vi "RSSI_Scanning.vi"() -> ()   [LabVIEW 2017]
uses:
  <vilib>/Instr/_visa.llb/VISA Configure Serial Port (Instr).vi
  Global Stop Variable.vi
  <vilib>/addons/_office/excel.llb/Excel Easy Table (str).vi
  <vilib>/Utility/NIReport.llb/NI_report.lvclass
  <vilib>/addons/_office/NI_ReportGenerationToolkit.lvlib
  <vilib>/Utility/NIReport.llb/Excel/NI_Excel.lvclass
panel:
  out "source":string
  out "code":i32
  out "error out":errorcluster
  out "STATUS":string
  in  "STOP":bool
  in  "Mode":T1(radio)
  out "Selesai Download":bool
  out "error out 2":errorcluster
  out "SSID 3":string
  out "SSID array":string[](array[string])
  out "dbm array":i32[](array[numeric])
  out "Color Box 3":u32(colorbox)=56508
  in  "Tab Control":T2(tab)
  in  "Tab Control 5":T3(tab)
  out "Background 8":string="Seiring dengan perkembangan teknologi informasi dan komunikasi yang pesat, jumlah pengguna internet di dunia mencapai 4,66 miliyar pada bulan januari tahun 2021 (Menurut hasil survey Hootsuite). Melihat data tersebut dapat disimpulkan bahwa akses internet sangat diminati dan menjadi kebutuhan utama oleh pengguna layanan internet [1]. Ada beberapa cara untuk mengakses internet yaitu dengan, Satellite, Celululer, Dial-Up, DSL, Cable, dan Wireless. WiFi, Berdasarkan IEEE 802.11 adalah sepesifikasi protokol jaringan lokal , dimana memungkinkan untuk mengakses internet dalam area yang terbatas menggunakan titik akses jaringan nirkabel atau dikenal dengan access point.  \nAccess point adalah perangkat jaringan yang berguna untuk membuat jaringan nirkabel yang sifatnya lokal dan berfungsi sebagai pintu gerbang bagi pengguna jaringan nirkabel untuk masuk ke dalam jaringan lokal.  Pada access point terdapat antena pengirim dan penerima sinyal, antena ini bertugas untuk memancarkan dan menerima sinyal dari clien server ataupun menuju clien server untuk bisa memancarkan sinyal WiFi. Dalam proses pengiriman dan penerimaan tersebut ada beberapa sistem untuk meningkatkan proses pengiriman dan penerimaan sinyal pada access point, yaitu menggunakan sistem MIMO pada access point, sehingga proses pengiriman dan penerimaan sinyal dapat meningkatkan kapasitas kanal atau jumlah aliran spasial [2][3].\n\nProses pengiriman dan penerimaan sinyal pada access point  dapat dilihat kekuatan sinyalnya dari parameter RSSI. Dalam literatur, [4] menyatakan bahwa RSSI merupakan parameter yang digunakan untuk mengukur indikator kekuatan sinyal yang diterima oleh sebuah access point. Dalam literatur, [5][6][7][8] parameter RSSI dimanfaatkan untuk membandingan kekuatan sinyal dan menganalisa hasil pengukuran RSSI terhadap access poin, jarak, dan ketinggian yang berbeda, dengan menggunakan perangkat lunak WiFi analyzer. Pada studi literatur tersebut terdapat dua kekurangan, yang pertama, dalam studi literatur terdahulu hanya menganalisa pengukuran RSSI terhadap variabel jarak dan tinggi terhadap acces point belum ada yang menganalisa pengukuran RSSI terhadap variabel polarisasi antena, dan yang kedua mengenai alat ukur yang digunakan oleh studi literatur, yaitu WiFi analyzer yang digunakan tidak memiliki fitur riwayat tercatat.\n\nBerdasarkan pemaparan di atas, maka dari itu diusulkan judul tugas akhir    \"Perancangan Wifi Analyzer Berbasis LabVIEW Untuk Membandingkan Parameter RSSI Pada Antena Access Point Sistem MIMO\".    Penelitian eksperimen ini diharapakan, pertama membuat alat ukur WiFi analyzer menggunakan NodeMCU  basis LabVIEW dengan fitur riwayat tercatat ke database, keterbukaan akses informasi dalam memperoleh parameter RSSI dan kemudahan komunikasi antar perangkat keras dengan perangkat lunak . Kedua, mengetahui ketepatan pengukuran kekuatan sinyal terima pada acces poin antena sistem MIMO menggunakan alat ukur yang telah dibuat. Ketiga, menganalisis pengaruh parameter RSSI dengan merubah variabel polarisasi pada antena access point sistem MIMO.\n\n"
  out "Background 7":string="Pemanas memiliki peran penting dalam proses industri, terutama industri kimia, yaitu untuk meningkatkan efisiensi proses dan menghasilkan kualitas produk yang baik. Salah satu jenis pemanas di industri kimia yang banyak digunakan adalah pemanas tangki berpengaduk. Pemanas tangki berpengaduk terdiri dari beberapa bagian, salah satunya adalah heater yang digunakan sebagai pemanas untuk mengubah bahan baku menjadi produk yang lebih bernilai guna. (N. I. Septiani, dkk, 2017)\n\nMasalah yang sering dihadapi dalam proses tersebut adalah keakuratan suhu pada tangki pemanas. Agar suhu tangki tersebut mencapai titik setel dengan kecepatan respons dan akurasi yang tinggi, maka diperlukan sebuah pengendali. (N. I. Septiani, dkk, 2017) Pengendali PID merupakan salah satu jenis pengendali yang paling banyak digunakan pada industri kimia dan industri yang memproduksi berbagai minuman seperti minuman coklat, susu, dan berbagai produk minuman lainnya. (A. Ramadhani, 2016) Untuk menghadapi tantangan industri tersebut, mahasiswa Diploma IV harus menguasai ilmu dan teknologi mengenai pengendali suhu pemanas tangki berpengaduk berbasis PID. \n\nMenurut Herman Dwi Surjono, media pembelajaran adalah program pembelajaran yang berisi teks, gambar, animasi, simulasi secara terpadu untuk mencapai tujuan pembelajaran. Media pembelajaran interaktif adalah program pembelajaran dimana pengguna secara aktif berinteraksi dengan program. Media pembelajaran interaktif memiliki ciri yaitu dapat mengontrol dan berinteraksi secara dinamis. Media pembelajaran interaktif dapat menumbuhkan pengalaman belajar melalui rangsangan visual, kesadaran afektif, penggalian informasi kognitif, dan pengembangan keterampilan psikomotorik. (H. Surjono, 2017)\n"
  out "Background 10":string="Proses pengiriman dan penerimaan sinyal pada access point  dapat dilihat kekuatan sinyalnya dari parameter Receiver Signal Strength Indicator ( RSSI ). Dalam literatur, [4] menyatakan bahwa RSSI merupakan parameter yang digunakan untuk mengukur indikator kekuatan sinyal yang diterima oleh sebuah access point. Dalam literatur, [5][6][7][8] parameter RSSI dimanfaatkan untuk membandingan kekuatan sinyal dan menganalisa hasil pengukuran RSSI terhadap access poin\n\nReceiver Signal Strength Indicator atau singkatan dari RSSI adalah istilah yang digunakan untuk mengukur kualitas relatif dari sinyal yang diterima ke perangkat wireless dan tidak memiliki nilai absolut. Standar IEEE 802.11 menetapkan bahwa RSSI dapat dalam skala 0 sampai dengan 255 dan bahwa masing-masing produsen chipset dapat menentukan nilai maksimumnya dia sendiri. Misalnya salah satu perusahaan network card menggunakan skala 0-100, sedangkan perusahaan lainnya menggunakan 0-60.\n\n\nhttps://rhiel.id/memahami-fitur-received-signal-strength-indication-rssi-pada-wireless-dan-implementasinya/"
  out "Background 9":string="Pemanas memiliki peran penting dalam proses industri, terutama industri kimia, yaitu untuk meningkatkan efisiensi proses dan menghasilkan kualitas produk yang baik. Salah satu jenis pemanas di industri kimia yang banyak digunakan adalah pemanas tangki berpengaduk. Pemanas tangki berpengaduk terdiri dari beberapa bagian, salah satunya adalah heater yang digunakan sebagai pemanas untuk mengubah bahan baku menjadi produk yang lebih bernilai guna. (N. I. Septiani, dkk, 2017)\n\nMasalah yang sering dihadapi dalam proses tersebut adalah keakuratan suhu pada tangki pemanas. Agar suhu tangki tersebut mencapai titik setel dengan kecepatan respons dan akurasi yang tinggi, maka diperlukan sebuah pengendali. (N. I. Septiani, dkk, 2017) Pengendali PID merupakan salah satu jenis pengendali yang paling banyak digunakan pada industri kimia dan industri yang memproduksi berbagai minuman seperti minuman coklat, susu, dan berbagai produk minuman lainnya. (A. Ramadhani, 2016) Untuk menghadapi tantangan industri tersebut, mahasiswa Diploma IV harus menguasai ilmu dan teknologi mengenai pengendali suhu pemanas tangki berpengaduk berbasis PID. \n\nMenurut Herman Dwi Surjono, media pembelajaran adalah program pembelajaran yang berisi teks, gambar, animasi, simulasi secara terpadu untuk mencapai tujuan pembelajaran. Media pembelajaran interaktif adalah program pembelajaran dimana pengguna secara aktif berinteraksi dengan program. Media pembelajaran interaktif memiliki ciri yaitu dapat mengontrol dan berinteraksi secara dinamis. Media pembelajaran interaktif dapat menumbuhkan pengalaman belajar melalui rangsangan visual, kesadaran afektif, penggalian informasi kognitif, dan pengembangan keterampilan psikomotorik. (H. Surjono, 2017)\n"
  out "Background 12":string="Pengertian Bandwidth\nSecara harfiah, bandwidth berarti ‘lebar pita’. Namun, makna sebenarnya juga tak jauh dari lebar pita ini. Dilansir dari ITPro, bandwidth pada dasarnya adalah jumlah data maksimum yang dapat ditransfer melalui koneksi internet selama periode waktu tertentu. Jadi, bandwidth ini mencakup kapasitas transmisi koneksi yang sangat penting dalam menentukan kualitas dan kecepatan koneksi internet.\n\nBandwidth ini diukur dalam satuan bit per second (bps) atau bit per detik. Biasanya kita sering mendengar istilah kecepatan Wi-Fi hingga 70 Mbps. Itu berarti, jaringan tersebut bisa mengirimkan data maksimal 70 MB per detik atau memiliki bandwidth 70 Mbps. Jaringan dengan bandwidth yang lebih tinggi dapat mentransfer lebih banyak data. Namun, perlu diingat bahwa bandwidth menandakan jumlah maksimal data yang dapat dikirim. Pada kenyataannya, sering kali jumlah ini tidak tercapai.\n\nBandwidth sering disamakan dengan kecepatan internet, padahal sebenarnya merupakan volume atau jumlah data yang dapat dikirim melalui koneksi dalam jumlah waktu tertentu. Cara kerja bandwidth ini sebenarnya masih sejalan dengan fungsinya sebagai media sekaligus pembatas untuk transfer data.\n\nSedangkan, Throughput adalah bandwidth yang aktual atau sebenarnya, yang diukur dengan satuan waktu tertentu dan pada kondisi jaringan tertentu yang digunakan untuk melakukan transfer data  dengan ukuran tertentu pula.\n\nDari gambar disamping menjelaskan bahwa, warna jingga yang merupakan bandwidth adalah lebar jalurnya. Sedangkan garis hitam yang merupakan throughput adalah kemampuan yang sebarnya yang mampu dibawa pada kondisi yang sebenarnya (aktual).\n\nJika misalnya bandwidth internet anda yang anda ketahui adalah 64 kbps, kemudian anda ingin mendownload file di Internet berukuran 128 kb, seharusnya file tersebut sudah sampai ke komputer anda hanya dengan waktu 2 detik (128/64).\n\nAkan tetapi  yang terjadi sebenarnya file yang anda download tiba dalam waktu 8 detik. Jadi bandwidth yang sebenarnya atau yang disebut throughtput adalah 128kb/8 detik = 16 kbps.\n\nhttps://www.acerid.com/apa-itu-bandwidth/\nhttps://www.selamatpagi.id/bandwidth-dan-throughput/\n\n"
  out "Background 11":string="Pemanas memiliki peran penting dalam proses industri, terutama industri kimia, yaitu untuk meningkatkan efisiensi proses dan menghasilkan kualitas produk yang baik. Salah satu jenis pemanas di industri kimia yang banyak digunakan adalah pemanas tangki berpengaduk. Pemanas tangki berpengaduk terdiri dari beberapa bagian, salah satunya adalah heater yang digunakan sebagai pemanas untuk mengubah bahan baku menjadi produk yang lebih bernilai guna. (N. I. Septiani, dkk, 2017)\n\nMasalah yang sering dihadapi dalam proses tersebut adalah keakuratan suhu pada tangki pemanas. Agar suhu tangki tersebut mencapai titik setel dengan kecepatan respons dan akurasi yang tinggi, maka diperlukan sebuah pengendali. (N. I. Septiani, dkk, 2017) Pengendali PID merupakan salah satu jenis pengendali yang paling banyak digunakan pada industri kimia dan industri yang memproduksi berbagai minuman seperti minuman coklat, susu, dan berbagai produk minuman lainnya. (A. Ramadhani, 2016) Untuk menghadapi tantangan industri tersebut, mahasiswa Diploma IV harus menguasai ilmu dan teknologi mengenai pengendali suhu pemanas tangki berpengaduk berbasis PID. \n\nMenurut Herman Dwi Surjono, media pembelajaran adalah program pembelajaran yang berisi teks, gambar, animasi, simulasi secara terpadu untuk mencapai tujuan pembelajaran. Media pembelajaran interaktif adalah program pembelajaran dimana pengguna secara aktif berinteraksi dengan program. Media pembelajaran interaktif memiliki ciri yaitu dapat mengontrol dan berinteraksi secara dinamis. Media pembelajaran interaktif dapat menumbuhkan pengalaman belajar melalui rangsangan visual, kesadaran afektif, penggalian informasi kognitif, dan pengembangan keterampilan psikomotorik. (H. Surjono, 2017)\n"
  in  "Tab Control 6":T4(tab)
  out "Background 20":string="/*\n    This sketch demonstrates how to scan WiFi networks.\n    The API is almost the same as with the WiFi Shield library,\n    the most obvious difference being the different file you need to include:\n*/\n#include <ESP8266WiFi.h>\n/*Fungsi void setup() dijalankan pada saat sketch atau program Arduino mulai.\nFungsi ini digunakan untuk menginisiasi variabel, mendeklarasikan pin yang digunakan,\nmenggunakan library, dll. */\nvoid setup() {\n  Serial.begin(115200);//buka port serial dengan bitrate 115200 baud\n  Serial.println(F(\"\\nESP8266 WiFi scan example\"));\n  // Set WiFi to station mode// station mode: the ESP32 connects to an access point\n  WiFi.mode(WIFI_STA);\n  // Disconnect from an AP if it was previously connected\n  WiFi.disconnect();\n  delay(100);\n}\n/*Fungsi void loop() dijalankan setelah fungsi setup() sudah selesai dijalankan,\n * void loop() bertujuan untuk mengeksekusi dan menjalankan program yang sudah dibuat.\nFungi ini akan secara aktif mengontrol board Arduino baik membaca input atau merubah output.\n*/ \nvoid loop() {\n  String ssid; /* String yaitu tipe data yang digunakan untuk menuliskan karakter atau teks,\n  bisa berupa huruf, angka atau karakter lain*/\n  int32_t RSSI; // mediumInt\n  uint8_t encryptionType; // smallInt\n  uint8_t* BSSID; // smallInt BSSID adalah nama lain dari SSID, SSID diberikan oleh pemakai misalnya “pcsaya” pada komputer yang sedang digunakan dan komputer lainnya dibuatkan nama “pckamu”. Sedangkan BSSID mengunakan basis MAC address.\n  int32_t channel; // mediumInt\n  bool isHidden;\n  int scanResult;\n/*Serial.print(\"This is a test - Hello world!!\");\nuses SRAM for the string, so few such prints and your SRAM is full.\nYou may use:\nSerial.print(F(\"This is a test - Hello world!!\"));\nand it uses FLASH for storing the string, thus you save the SRAM.\np.*/\n  Serial.println(F(\"Starting WiFi scan...\"));\n  scanResult = WiFi.scanNetworks();\n  \n  if (scanResult == 0) {\n    Serial.println(F(\"No networks found\"));\n  } else if (scanResult > 0) {\n    Serial.printf(PSTR(\"%d networks found:\\n\"), scanResult);\n\n    // Print unsorted scan results\n    for (int8_t i = 0; i < scanResult; i++) {\n      WiFi.getNetworkInfo(i, ssid, encryptionType, RSSI, BSSID, channel, isHidden);\n// %02d : dua digit\n      Serial.printf(PSTR(\"  %02d: [CH %02d] [%02x:%02x:%02x:%02x:%02x:%02x] %ddBm %c %c %s\\n\"),\n                    i, channel, BSSID[0], BSSID[1], BSSID[2], BSSID[3], BSSID[4], BSSID[5], RSSI,\n                    (encryptionType == ENC_TYPE_NONE) ? ' ' : '*',\n                    isHidden ? 'H' : 'V',\n                    ssid.c_str());\n      delay(0);\n    }\n  } else {\n    Serial.printf(PSTR(\"WiFi scan error %d\"), scanResult);\n  }\n\n  // Wait a bit before scanning again\n  delay(5000);\n}"
  out "Background 19":string="1.Buka Arduino IDE\n\n2.Copy dan Paste program arduino RSSI yang     terdapat pada indicator box Program Arduino\n\n3.Sambungakan USB ke nodeMcu dan personal komputer atau laptop\n\n4.Atur board NodeMcu 1.0 (ESP-12E Module)\nAtur port USB nodeMcu\n\n5.Compile program arduino RSSI\n\n6.Upload Program\n\n7.Buka serial monitor\n\n8.masukan baudrade 115200\n\n9.setelah datanya keluar berarti indikator program berhasil diupload ke nodeMcu\n\n10.kemudian close serial monitor arduino IDE\n\n11.Buka Software LabVIEW\n\n12.Jalankan program labview\n\n13.Pahami penggunaan program RSSI pada LabVIEW dengan membaca alur diagram prinsip kerja RSSI di sebelah kanan\n\n14.Pastiakan terhubung ke jaringan internet untuk menjalankan mode troughput\n\nPastikan akses internet ketika menggunkan mode troughput\n\n\n"
  out "Background 14":string=">Perangkat Lunak\n1.Install Arduino IDE\n2.Install Board nodeMcu pada Arduino IDE\n- http://arduino.esp8266.com/stable/package_esp8266com_index.json\n3.Paste Library wifi scan ke directory Arduino IDE\n- https://github.com/esp8266/Arduino/blob/master/libraries/ESP8266WiFi/examples/WiFiScan/WiFiScan.ino\n4.Install driver CH341 pada Ardunio IDE\n5.Install Labview 2017\n6.Install driver niserial1700f0\n7.Install library WiFi di vi package manager\n- https://forums.ni.com/t5/Example-Code/WiFi-Network-Scanning-and-Connecting-with-LabVIEW/ta-p/3731977?profile.language=en\n\n>Perangkat Keras\n1.Menggunakan NodeMcu\n2.Menggunakan Micro USB 2.0 Cable"
  out "Background 13":string="Pemanas memiliki peran penting dalam proses industri, terutama industri kimia, yaitu untuk meningkatkan efisiensi proses dan menghasilkan kualitas produk yang baik. Salah satu jenis pemanas di industri kimia yang banyak digunakan adalah pemanas tangki berpengaduk. Pemanas tangki berpengaduk terdiri dari beberapa bagian, salah satunya adalah heater yang digunakan sebagai pemanas untuk mengubah bahan baku menjadi produk yang lebih bernilai guna. (N. I. Septiani, dkk, 2017)\n\nMasalah yang sering dihadapi dalam proses tersebut adalah keakuratan suhu pada tangki pemanas. Agar suhu tangki tersebut mencapai titik setel dengan kecepatan respons dan akurasi yang tinggi, maka diperlukan sebuah pengendali. (N. I. Septiani, dkk, 2017) Pengendali PID merupakan salah satu jenis pengendali yang paling banyak digunakan pada industri kimia dan industri yang memproduksi berbagai minuman seperti minuman coklat, susu, dan berbagai produk minuman lainnya. (A. Ramadhani, 2016) Untuk menghadapi tantangan industri tersebut, mahasiswa Diploma IV harus menguasai ilmu dan teknologi mengenai pengendali suhu pemanas tangki berpengaduk berbasis PID. \n\nMenurut Herman Dwi Surjono, media pembelajaran adalah program pembelajaran yang berisi teks, gambar, animasi, simulasi secara terpadu untuk mencapai tujuan pembelajaran. Media pembelajaran interaktif adalah program pembelajaran dimana pengguna secara aktif berinteraksi dengan program. Media pembelajaran interaktif memiliki ciri yaitu dapat mengontrol dan berinteraksi secara dinamis. Media pembelajaran interaktif dapat menumbuhkan pengalaman belajar melalui rangsangan visual, kesadaran afektif, penggalian informasi kognitif, dan pengembangan keterampilan psikomotorik. (H. Surjono, 2017)\n"
  out "Log Window":string
  in  "Connect":bool
  in  "Network":i32(ring) items=["Yul-MiFi 2", "Yul-MiFi", "BANDUNG LAUTAN API", "KAMAR206", "Rumahku", "almamaula", "WiFi.id"]
  in  "Tab Control 2":enum32{"Export To Data Base", "Troughput"}(tab)
  in  "Header Caption":string
  in  "dbm position":cluster{"row":i32, "column":i32}={"row"=2, "column"=1}
  in  "SSID Poisition":cluster{"row":i32, "column":i32}={"row"=2, "column"=0}
  in  "DatBase":bool
  in  "URL":string
  in  "Path":path
  out "Size (in bytes)":i64
  out "Second":dbl
  out "Mb/s":dbl
  in  "Download":bool
  in  "Show File in Explorer":bool=TRUE
  out "Downloading":bool
  out "Finish":bool
  out "Error":bool
  out "Hystorical":string[][](table)
  out "1":string
  out "2":string
  out "3":string
  out "4":string
  out "5":string
  out "6":string
  out "Channel":i32
  out "Encrytion":string
  out "Is Hidden":string
  in  "Select Port":refnum<visa-resource-name>
  out "Read Buffer":string
  out "SSID":string
  out "dbm":i32
  out "No":i32
  out "Color Box 4":u32(colorbox)=11918273
  out "Color Box 5":u32(colorbox)=11918273
  # "Alur Diagram Prinsip Kerja Program RSSI"
  # "WiFi Analyzer Berbasis LabVIEW"
  # "Dodi Kusuma (2021), Politeknik Manufaktur Bandung: Teknologi Rekayasa Otomasi"
  # "Select Menu"
  # "STOP"
  # "Test troughput\n- sub vi harus kebuka\n- link downloadnya jangan panjang nanti error\n- error kalau ada proses login nya\n- download file rar belum ada\n- error download python\n- stop global gak bisa berfungsi ketika downloading sedang berlangsung\n   ( sub vi download tetap running )\n- tombol downloadnya masih belum stabil\n- kalau dari mode troughput pindah ke yg lain scanning lanjut tidak mulai dari awal\n- jumlah SSID nya tidak diperbaruhi ( WIFI Library )"
  # "Scaning RSSI"
  # "Export  to Data Base"
  # "Troughput Testing"
  # "Latar Belakang"
  # "Latar Belakang"
  # "RSSI"
  # "Latar Belakang"
  # "Rumus RSSI (dBm)"
  # "Troughput"
  # "Latar Belakang"
  # "Perbedaan Bandwidht dan Troughput"
  # "Rumus"
  # "Latar Belakang"
  # "Latar Belakang"
  # "Developed By\nDodi Kusuma\n\nEmail: 1. dodi.mahasiswa@mhs.polman-bandung.ac.id\n2. dodykusuma98@gmail.com\n\nUpdated  12 July 2020 \nDeveloped in LabVIEW 2017"
  # "Komponen Pendukung"
  # "Latar Belakang"
  # "Prosedur Penggunaan Software"
  # "Program Arduino"
  # "Latar Belakang"
  # "Latar Belakang"
  # "Developed By\nDodi Kusuma\n\nEmail: 1. dodi.mahasiswa@mhs.polman-bandung.ac.id\n2. dodykusuma98@gmail.com\n\nUpdated  12 July 2020 \nDeveloped in LabVIEW 2017"
  # "Package Information"
  # "BSSID"
  # "Scrool the monitor screen"
  # "Temporary historical"
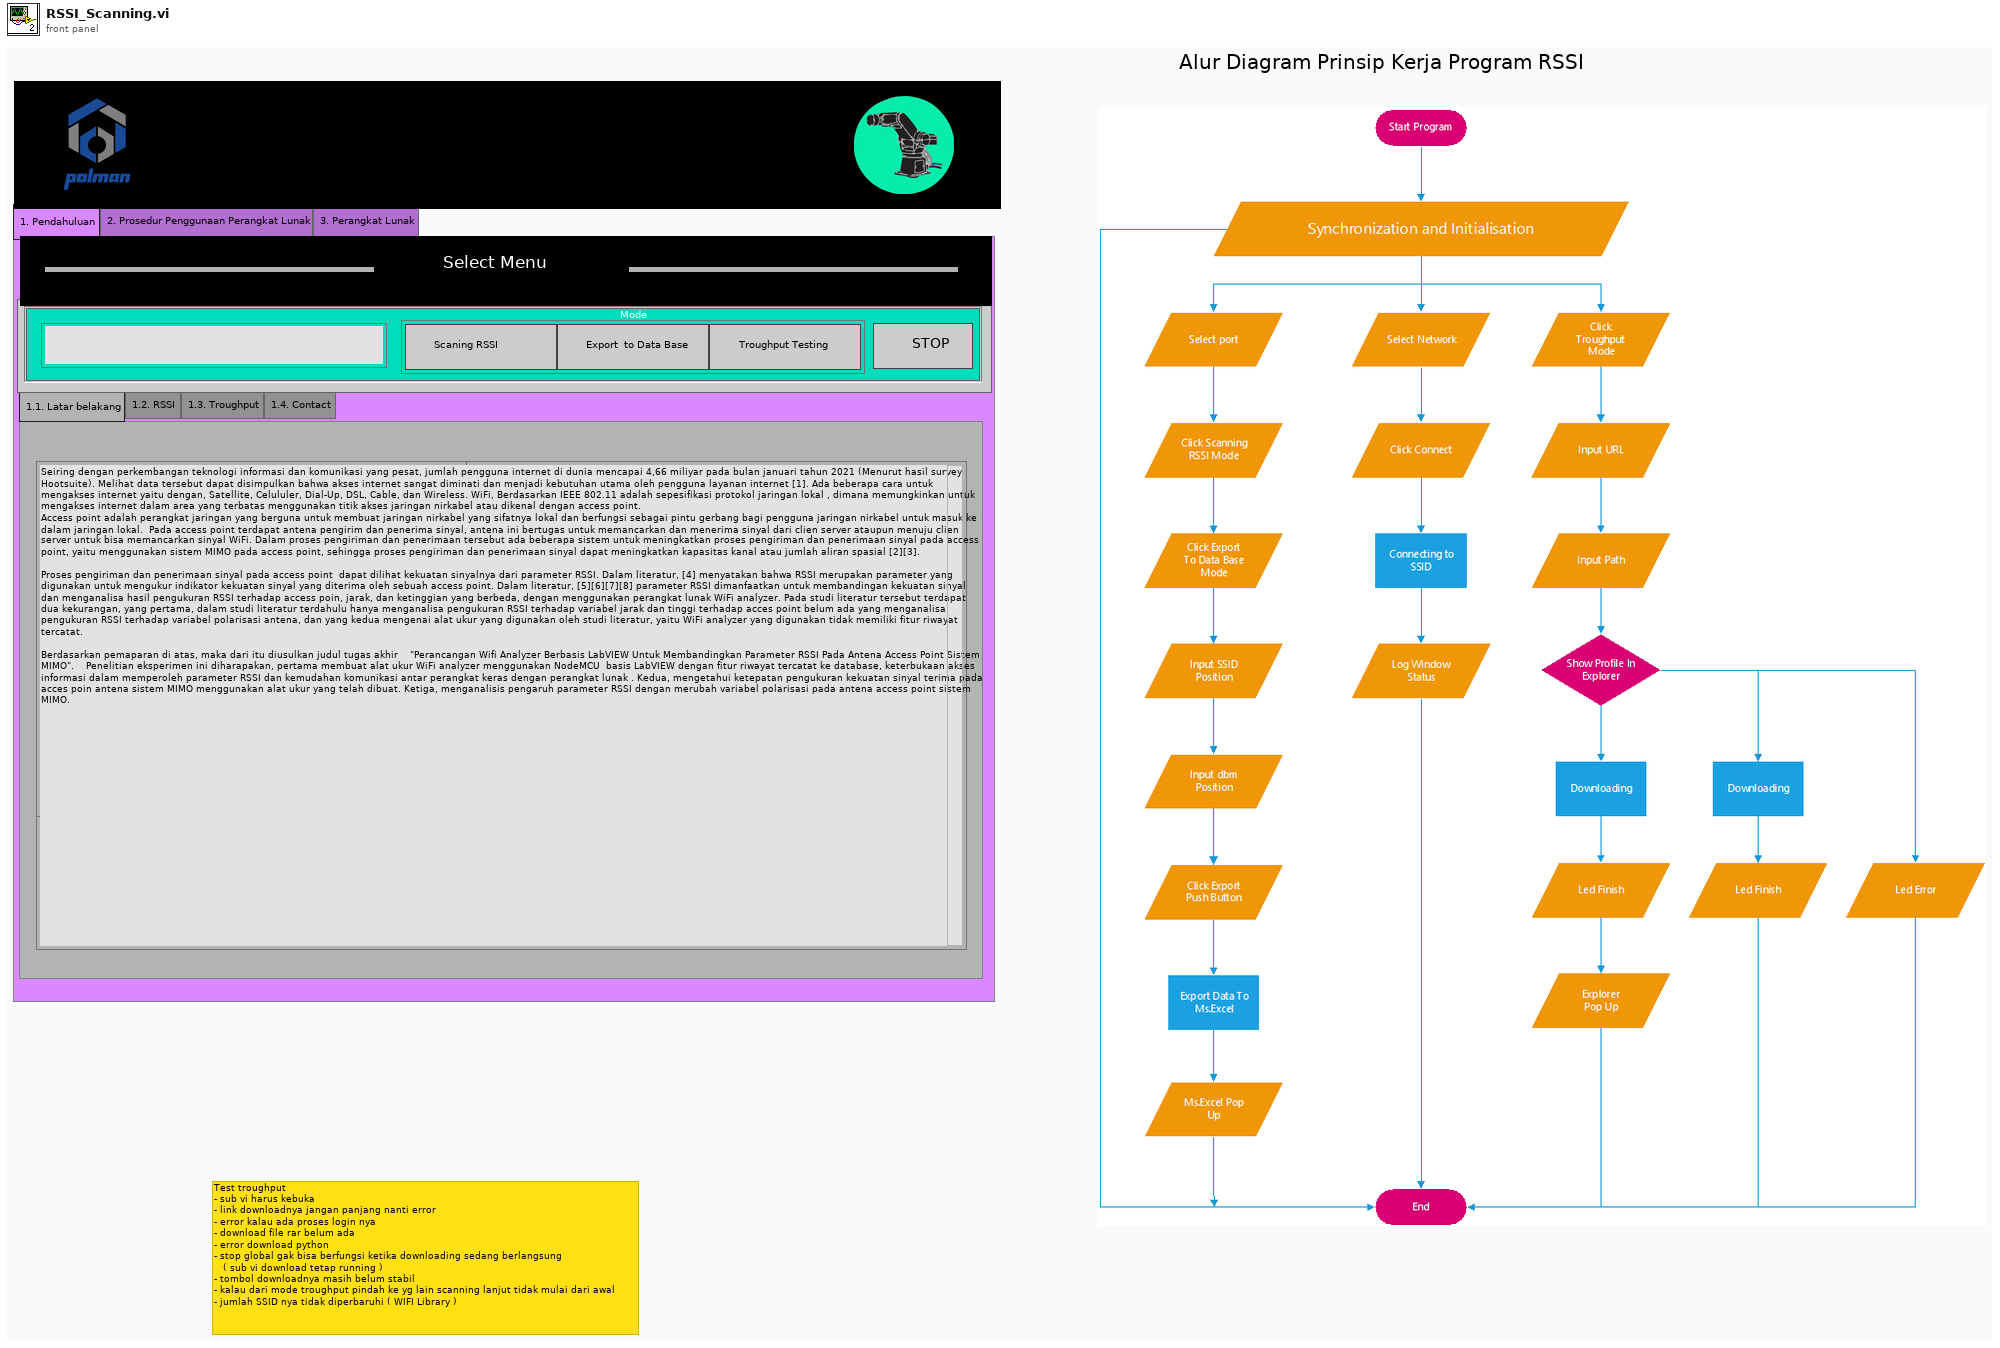
[diagram p1: front panel]
types:
  T1 = enum32{"No Selection", "RRSI Mode", "Data Base Mode", "Troughput Mode"}
  T2 = enum32{"1. Pendahuluan", "2. Prosedur Penggunaan Perangkat Lunak", "3. Perangkat Lunak"}
  T3 = enum32{"1.1. Latar belakang", "1.2. RSSI", "1.3. Troughput", "1.4. Contact"}
  T4 = enum32{"1.1. Syarat dan Prosedur", "1.4. Contact"}
  T5 = cluster{"on/off":bool, "weight":i32, "color":u32}
  T6 = enum16{"Standard Report", "HTML", "Word", "Excel"}
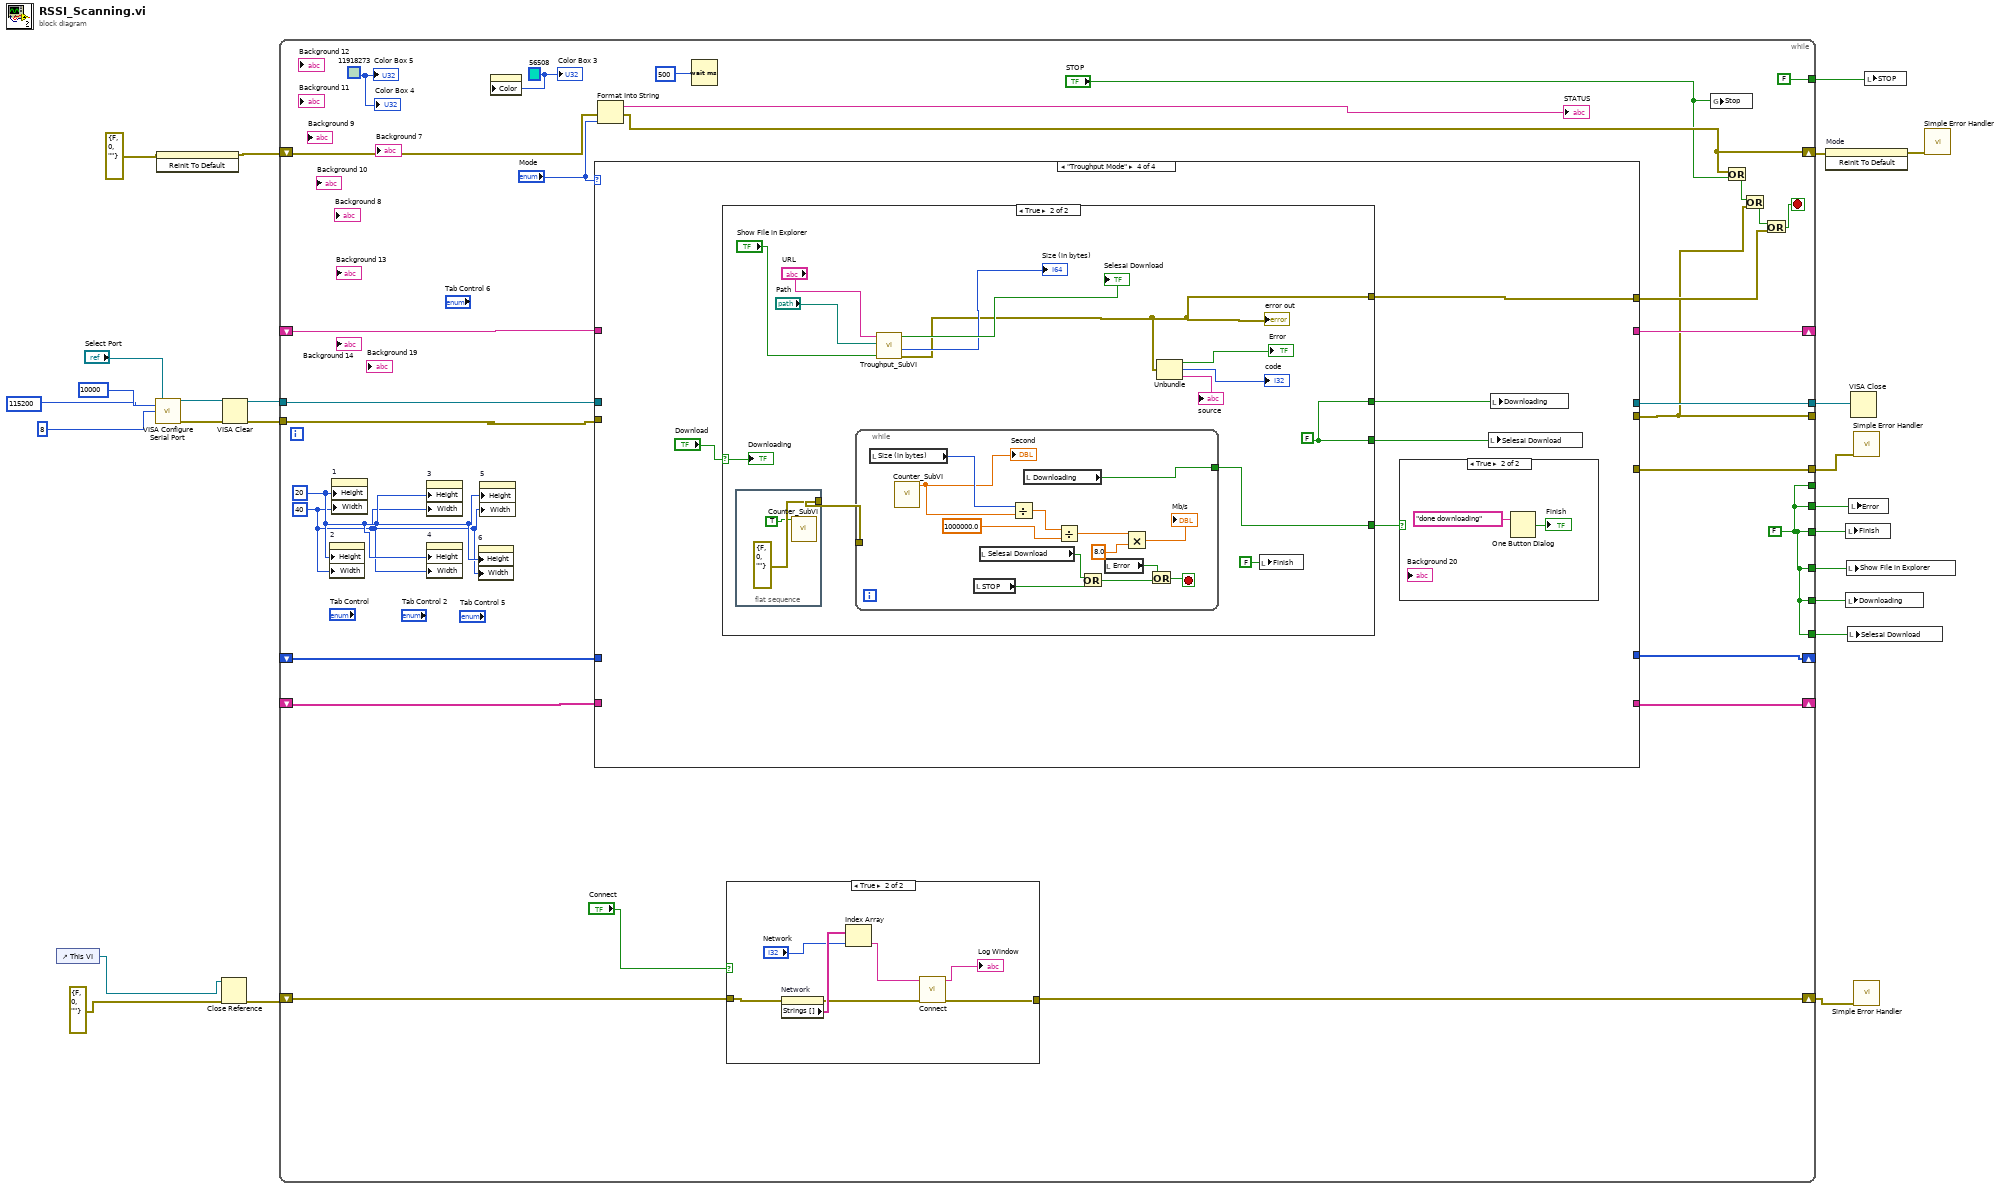
[diagram p0: block diagram]
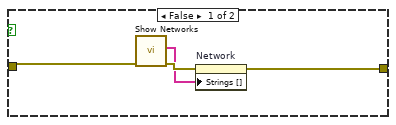
[diagram p2: hidden frame]
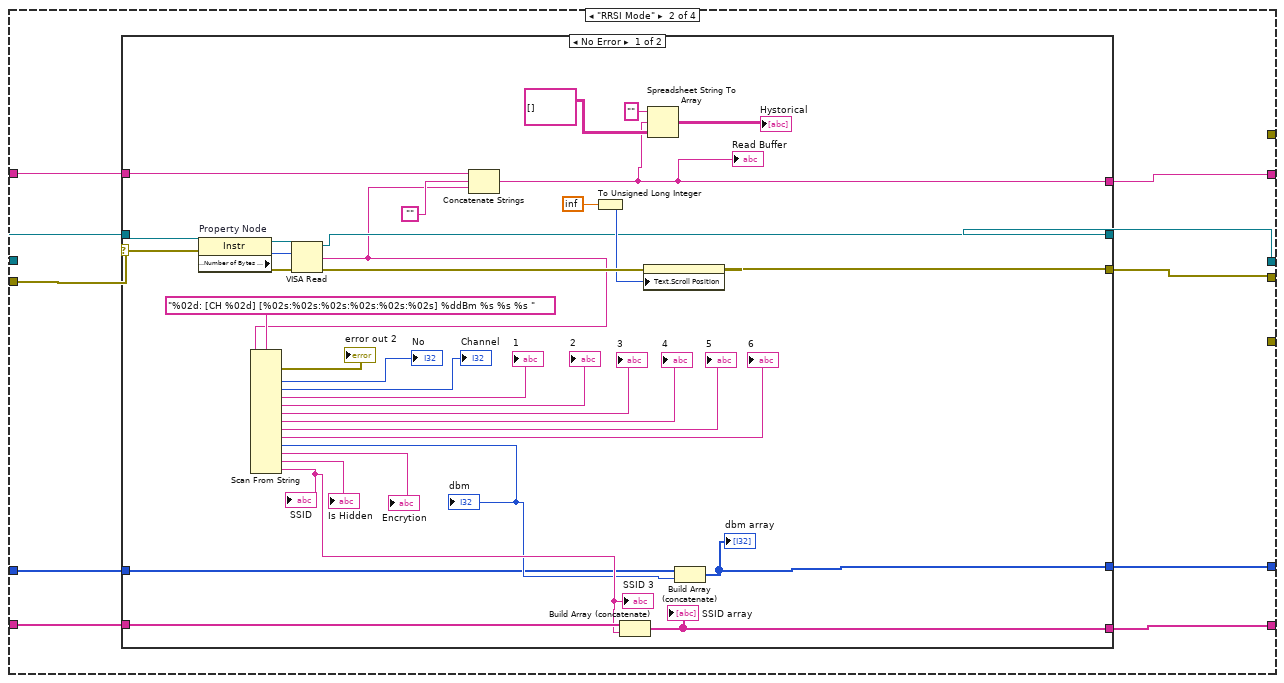
[diagram p4: hidden frame]
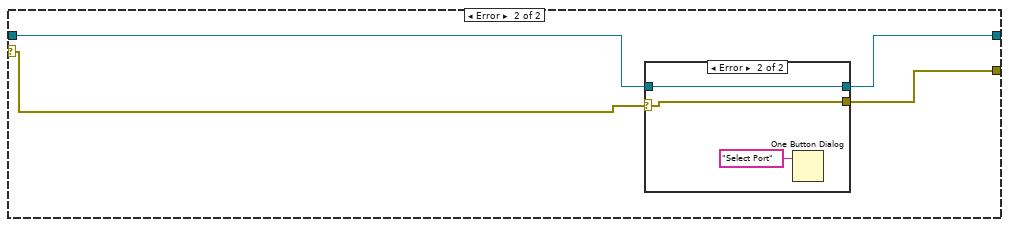
[diagram p5: hidden frame]
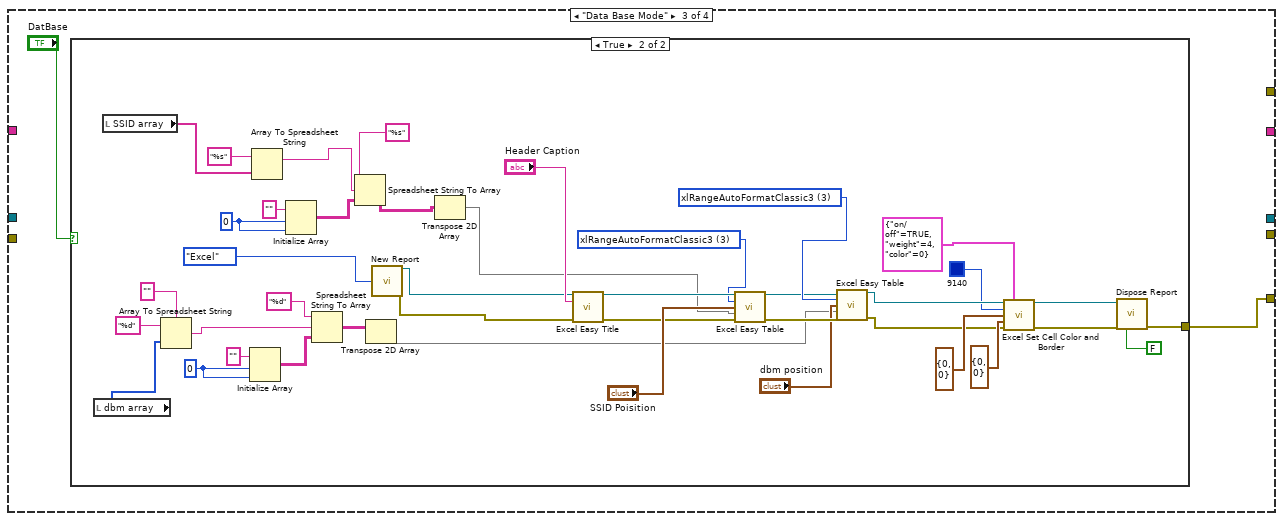
[diagram p7: hidden frame]
diagram:
  n1 = control-ref of="This VI"() -> (w2:refnum<vi>)
  n2 = call-poly "VISA Configure Serial Port"("VISA resource name"="Select Port", "timeout (10sec)"=u32 10000, "baud rate (9600)"=u32 115200, "data bits (8)"=u16 8) -> ("VISA resource name out"=w17:refnum<visa-resource-name>, "error out"=w16:errorcluster)  [unwired: 10 in]
  n3 = invoke on="Mode" class="RadioBtnsControl (strict)" method="Reinit To Default"(error in=errorcluster {"status"=FALSE, "code"=0, "source"=""} ("error constant")) -> (error out=w23:errorcluster)  [unwired: 2 in, 2 out]
  n4 = Close Reference(reference=w2, error in (no error)=errorcluster {"status"=FALSE, "code"=0, "source"=""} ("error out")) -> (error out=w4:errorcluster)
  n5 = VISA Clear(VISA resource name=w17, error in (no error)=w16) -> (VISA resource name out=w15:refnum<visa-resource-name>, error out=w14:errorcluster)
  n6 = while {
    shift-right: [w48] -> w10
    shift-left: w23 -> [w49]
    tunnel: [w53] -> w18
    shift-right: [w44] -> _
    shift-left: _ -> [w46]
    shift-right: [w45] -> _
    shift-left: _ -> [w47]
    shift-right: [w43] -> _
    shift-left: _ -> [w35]
    tunnel: w15 -> [w52]
    tunnel: w14 -> [w40]
    tunnel: [w32] -> _
    tunnel: [w31] -> w13
    tunnel: [FALSE ("STOP")] -> w12
    tunnel: [w27] -> w11
    tunnel: [w27] -> w8
    tunnel: [w27] -> w7
    tunnel: [w27] -> w6
    tunnel: [w27] -> w5
    shift-right: [w25] -> w3
    shift-left: w4 -> [w28]
    tunnel: [w27] -> _
    stop <- w41 stop-if-true
    w27 = FALSE ("Finish")
    w37 = u32 56508 ("Color Box")
    w36 = u32 11918273 ("Color Box")
    w38 = u32 40 ("Size:Width")
    w39 = u32 20 ("Size:Height")
    n7 = property on="2" class="Str"("Height"=w39, "Width"=w38) -> ()  [unwired: 2 in, 2 out]
    n8 = property on="1" class="Str"("Height"=w39, "Width"=w38) -> ()  [unwired: 2 in, 2 out]
    n9 = property on="3" class="Str"("Height"=w39, "Width"=w38) -> ()  [unwired: 2 in, 2 out]
    n10 = property on="4" class="Str"("Height"=w39, "Width"=w38) -> ()  [unwired: 2 in, 2 out]
    n11 = property on="6" class="Str"("Height"=w39, "Width"=w38) -> ()  [unwired: 2 in, 2 out]
    n12 = property on="5" class="Str"("Height"=w39, "Width"=w38) -> ()  [unwired: 2 in, 2 out]
    n13 = property on="Mode" class="RadioBtnsControl (strict)"("Color"=w37) -> ()  [unwired: 2 in, 2 out]
    n14 = case shown="\"Troughput Mode\"" "Mode" {
      tunnel: [_ w74 _ _] -> w53
      tunnel: w52 -> [_ w75 _ _]
      tunnel: w40 -> [_ w66 _ _]
      tunnel: [_ w73 _ _] -> w32
      tunnel: w47 -> [_ w72 _ _]
      tunnel: w46 -> [_ w71 _ _]
      tunnel: [_ w70 _ _] -> w45
      tunnel: [_ w69 _ _] -> w44
      tunnel: w35 -> [_ w68 _ _]
      tunnel: [_ w67 _ _] -> w43
      tunnel: [_ _ _ w166] -> w42
      tunnel: [_ _ w120 _] -> w31
      frame "No Selection", Default {
      }
      frame "RRSI Mode" {
        n15 = case shown="No Error" w66 {
          selector: w66 -> [w91 w114]
          tunnel: w75 -> [w92 w112]
          tunnel: [w90 w111] -> w74
          tunnel: [w81 w113] -> w73
          tunnel: w71 -> [w89 _]
          tunnel: w72 -> [w86 _]
          tunnel: [w76 _] -> w70
          tunnel: [w83 _] -> w69
          tunnel: [w78 _] -> w67
          tunnel: w68 -> [w82 _]
          frame No Error {
            n16 = property on="Property Node" class="Instr"(reference=w92, error in=w91) -> (reference out=w110:refnum<visa-resource-name>, error out=w109:errorcluster, "Serial Settings:Number of Bytes at Serial Port"=w108:u32)
            n17 = VISA Read(VISA resource name=w110, byte count=w108, error in (no error)=w109) -> (VISA resource name out=w90:refnum<visa-resource-name>, read buffer=w84:string, error out=w101:errorcluster)  [unwired: 1 out]
            n18 = Scan From String(format string="%02d: [CH %02d] [%02s:%02s:%02s:%02s:%02s:%02s] %ddBm %s %s %s ", input string=w84) -> (error out=→"error out 2":errorcluster, output 1=→"No":i32, output 2=→"Channel":i32, output 3=→"1":string, output 4=→"2":string, output 5=→"3":string, output 6=→"4":string, output 7=→"5":string, output 8=→"6":string, output 9=w87:i32, output 10=→"Encrytion":string, output 11=→"Is Hidden":string, output 12=w88:string)  [unwired: 14 in, 2 out]
            "dbm" <- w87
            "SSID" <- w88
            "SSID 3" <- w88
            n19 = Concatenate Strings(w82, "", w84) -> (w78:string)
            "Read Buffer" <- w78
            n20 = To Unsigned Long Integer(number=inf) -> (unsigned 32bit integer=w93:u32)
            n21 = Build Array (concatenate)(w89, w88) -> (w83:string[])
            "SSID array" <- w83
            n22 = property class="Str"(error in=w101, "Text.Scroll Position"=w93) -> (error out=w81:errorcluster)  [unwired: 1 in, 1 out]
            n23 = Spreadsheet String To Array(format string="", spreadsheet string=w78, array type (2D Dbl)=string[][] [] ("Array")) -> (array=→"Hystorical":string[][])  [unwired: 1 in]
            n24 = Build Array (concatenate)(w86, w87) -> (w76:i32[])
            "dbm array" <- w76
          }
          frame Error {
            n25 = case shown="Error" w114 {
              selector: w114 -> [_ w117]
              tunnel: [_ w117] -> w113
              tunnel: w112 -> [w115 w116]
              tunnel: [w115 w116] -> w111
              frame No Error {
              }
              frame Error {
                n26 = One Button Dialog(message="Select Port") -> ()  [unwired: 1 in, 1 out]
              }
            }
          }
        }
      }
      frame "Data Base Mode" {
        n27 = case shown="True" "DatBase" {
          tunnel: [_ w138] -> w120
          frame False {
          }
          frame True {
            w137 = 3 items=["xlRangeAutoFormat3DEffects1"=13, "xlRangeAutoFormat3DEffects2"=14, "xlRangeAutoFormatAccounting1"=4, "xlRangeAutoFormatAccounting2"=5, "xlRangeAutoFormatAccounting3"=6, "xlRangeAutoFormatAccounting4"=17, "xlRangeAutoFormatClassic1"=1, "xlRangeAutoFormatClassic2"=2, "xlRangeAutoFormatClassic3"=3, "xlRangeAutoFormatColor1"=7, "xlRangeAutoFormatColor2"=8, "xlRangeAutoFormatColor3"=9, "xlRangeAutoFormatList1"=10, "xlRangeAutoFormatList2"=11, "xlRangeAutoFormatList3"=12, "xlRangeAutoFormatLocalFormat1"=15, "xlRangeAutoFormatLocalFormat2"=16, "xlRangeAutoFormatLocalFormat3"=19, "xlRangeAutoFormatLocalFormat4"=20, "xlRangeAutoFormatReport1"=21, "xlRangeAutoFormatReport2"=22, "xlRangeAutoFormatReport3"=23, "xlRangeAutoFormatReport4"=24, "xlRangeAutoFormatReport5"=25, "xlRangeAutoFormatReport6"=26, "xlRangeAutoFormatReport7"=27, "xlRangeAutoFormatReport8"=28, "xlRangeAutoFormatReport9"=29, "xlRangeAutoFormatReport10"=30, "xlRangeAutoFormatClassicPivotTable"=31, "xlRangeAutoFormatTable1"=32, "xlRangeAutoFormatTable2"=33, "xlRangeAutoFormatTable3"=34, "xlRangeAutoFormatTable4"=35, "xlRangeAutoFormatTable5"=36, "xlRangeAutoFormatTable6"=37, "xlRangeAutoFormatTable7"=38, "xlRangeAutoFormatTable8"=39, "xlRangeAutoFormatTable9"=40, "xlRangeAutoFormatTable10"=41, "xlRangeAutoFormatPTNone"=42, "xlRangeAutoFormatNone"=-4142, "xlRangeAutoFormatSimple"=-4154] ("auto format")
            w142 = 3 items=["xlRangeAutoFormat3DEffects1"=13, "xlRangeAutoFormat3DEffects2"=14, "xlRangeAutoFormatAccounting1"=4, "xlRangeAutoFormatAccounting2"=5, "xlRangeAutoFormatAccounting3"=6, "xlRangeAutoFormatAccounting4"=17, "xlRangeAutoFormatClassic1"=1, "xlRangeAutoFormatClassic2"=2, "xlRangeAutoFormatClassic3"=3, "xlRangeAutoFormatColor1"=7, "xlRangeAutoFormatColor2"=8, "xlRangeAutoFormatColor3"=9, "xlRangeAutoFormatList1"=10, "xlRangeAutoFormatList2"=11, "xlRangeAutoFormatList3"=12, "xlRangeAutoFormatLocalFormat1"=15, "xlRangeAutoFormatLocalFormat2"=16, "xlRangeAutoFormatLocalFormat3"=19, "xlRangeAutoFormatLocalFormat4"=20, "xlRangeAutoFormatReport1"=21, "xlRangeAutoFormatReport2"=22, "xlRangeAutoFormatReport3"=23, "xlRangeAutoFormatReport4"=24, "xlRangeAutoFormatReport5"=25, "xlRangeAutoFormatReport6"=26, "xlRangeAutoFormatReport7"=27, "xlRangeAutoFormatReport8"=28, "xlRangeAutoFormatReport9"=29, "xlRangeAutoFormatReport10"=30, "xlRangeAutoFormatClassicPivotTable"=31, "xlRangeAutoFormatTable1"=32, "xlRangeAutoFormatTable2"=33, "xlRangeAutoFormatTable3"=34, "xlRangeAutoFormatTable4"=35, "xlRangeAutoFormatTable5"=36, "xlRangeAutoFormatTable6"=37, "xlRangeAutoFormatTable7"=38, "xlRangeAutoFormatTable8"=39, "xlRangeAutoFormatTable9"=40, "xlRangeAutoFormatTable10"=41, "xlRangeAutoFormatPTNone"=42, "xlRangeAutoFormatNone"=-4142, "xlRangeAutoFormatSimple"=-4154] ("auto format")
            w154 = 0 ("dimension size")
            w156 = 0 ("dimension size")
            n28 = local read "dbm array"() -> (w122:i32[])
            n29 = local read "SSID array"() -> (w148:string[])
            n30 = Array To Spreadsheet String(delimiter (Tab)="", array=w122, 3:"%d" ("format string")) -> (spreadsheet string=w147:string)
            n31 = Initialize Array("" ("element"), w154, w154) -> (w159:string[][])
            n32 = Array To Spreadsheet String(array=w148, 3:"%s" ("format string")) -> (spreadsheet string=w131:string)  [unwired: 1 out]
            n33 = Initialize Array("" ("element"), w156, w156) -> (w161:string[][])
            n34 = Spreadsheet String To Array(format string="%d", spreadsheet string=w147, array type (2D Dbl)=w159) -> (array=w158:string[][])  [unwired: 1 out]
            n35 = Spreadsheet String To Array(format string="%s", spreadsheet string=w131, array type (2D Dbl)=w161) -> (array=w160:string[][])  [unwired: 1 out]
            n36 = Transpose 2D Array(2D array=w158) -> (transposed array=w132:string[][])
            n37 = call <vilib>:"New Report.vi"("report type"=T6."Excel") -> ("report out"=w141:refnum<class "NI_report.lvclass">, "error out"=w140:errorcluster)  [unwired: 13 in]
            n38 = Transpose 2D Array(2D array=w160) -> (transposed array=w133:string[][])
            n39 = call <vilib>:"Excel Easy Title.vi"("report in"=w141, "title"="Header Caption", "error in (no error)"=w140) -> ("report out"=w143:refnum<class "NI_report.lvclass">, "error out"=w144:errorcluster)  [unwired: 10 in, 1 out]
            n40 = call-poly <vilib>:"Excel Easy Table.vi"("report in"=w143, "auto format (none)"=w142, "start (0, 0)"="SSID Poisition", "text data"=w133, "error in (no error)"=w144) -> ("report out"=w136:refnum<class "NI_report.lvclass">, "error out"=w135:errorcluster)  [unwired: 6 in, 3 out]
            n41 = call-poly <vilib>:"Excel Easy Table.vi"("report in"=w136, "auto format (none)"=w137, "start (0, 0)"="dbm position", "text data"=w132, "error in (no error)"=w135) -> ("report out"=w127:refnum<class "NI_report.lvclass">, "error out"=w128:errorcluster)  [unwired: 6 in, 3 out]
            n42 = call <vilib>:"Excel Set Cell Color and Border.vi"("report in"=w127, "inside border"=T5 {"on/off"=TRUE, "weight"=4, "color"=0}, "background color (w)"=u32 9140, "start (-1, -1)"=cluster{"row":i32, "column":i32} {"row"=0, "column"=0}, "end (-1, -1)"=cluster{"row":i32, "column":i32} {"row"=0, "column"=0}, "error in (no error)"=w128) -> ("report out"=w126:refnum<class "NI_report.lvclass">, "error out"=w125:errorcluster)  [unwired: 8 in]
            n43 = call-dynamic "Dispose Report.vi"("report in"=w126, "error in (no error)"=w125, "close report? (T)"=FALSE ("Close Report? (T)")) -> ("error out"=w138:errorcluster)  [unwired: 12 in]
          }
        }
      }
      frame "Troughput Mode" {
        n44 = case shown="True" "Download" {
          selector: "Download" -> [_ w169]
          tunnel: [_ w170] -> w166
          tunnel: [_ w181] -> w165
          tunnel: [_ w181] -> w164
          tunnel: [_ w177] -> w162
          frame False {
          }
          frame True {
            w181 = FALSE ("Done")
            n45 = flat-sequence {
              tunnel: [errorcluster {"status"=FALSE, "code"=0, "source"=""} ("error constant")] -> w182
              frame #0 {
                n46 = call "Counter_SubVI.vi"("s"=TRUE) -> ()  [unwired: 9 in, 1 out]
              }
            }
            n47 = while {
              tunnel: w182 -> [_]
              tunnel: [w188] -> w177
              stop <- w186 stop-if-true
              n48 = local read "Size (in bytes)"() -> (w192:i64)
              n49 = call "Counter_SubVI.vi"() -> ("t"=w191:dbl)  [unwired: 10 in]
              "Second" <- w191
              n50 = local read "STOP"() -> (w189:bool)
              n51 = local read "Selesai Download"() -> (w190:bool)
              n52 = Divide(x=w192, y=w191) -> (x/y=w197:dbl)
              n53 = local read "Downloading"() -> (w188:bool)
              n54 = Divide(x=w197, y=1000000.0 ("x")) -> (x/y=w194:dbl)
              n55 = Or(x=w190, y=w189) -> (x .or. y?=w187:bool)
              n56 = local read "Error"() -> (w185:bool)
              n57 = Multiply(x=w194, y=8.0) -> (x*y=→"Mb/s":dbl)
              n58 = Or(x=w185, y=w187) -> (x .or. y?=w186:bool)
            }
            n59 = call "Troughput_SubVI.vi"("Show File in Explorer"="Show File in Explorer", "path"="Path", "URL"="URL") -> ("error out"=w170:errorcluster, "size (in bytes)"=→"Size (in bytes)":i64, "Indicator"=→"Selesai Download":bool)  [unwired: 6 in]
            "error out" <- w170
            n60 = Unbundle(w170) -> ("status"=→"Error":bool, "code"=→"code":i32, "source"=→"source":string)
            n61 = local write "Finish"(FALSE ("Finish")) -> ()
            "Downloading" <- w169
          }
        }
        n62 = case shown="True" w162 {
          frame False {
          }
          frame True {
            n63 = One Button Dialog(message="done downloading") -> (true=→"Finish":bool)  [unwired: 1 in]
          }
        }
        n64 = local write "Selesai Download"(w165) -> ()
        n65 = local write "Downloading"(w164) -> ()
      }
    }
    n66 = Format Into String(error in=w49, "Mode") -> (resulting string=→"STATUS":string, error out=w48:errorcluster)  [unwired: 2 in]
    n67 = Wait (ms)(milliseconds to wait=u32 500) -> ()  [unwired: 1 out]
    n68 = case shown="True" "Connect" {
      tunnel: [w58 w65] -> w25
      tunnel: w28 -> [w56 w64]
      frame False {
        n69 = call <userlib>:"Show Networks.vi"("error in (no error)"=w56) -> ("error out"=w57:errorcluster, "SSID"=w55:string[])  [unwired: 8 in, 1 out]
        n70 = property on="Network" class="Ring (strict)"(error in=w57, "Strings []"=w55) -> (error out=w58:errorcluster)  [unwired: 1 in, 1 out]
      }
      frame True {
        n71 = property on="Network" class="Ring (strict)"(error in=w64) -> (error out=w62:errorcluster, "Strings []"=w63:string[])  [unwired: 1 in, 1 out]
        n72 = Index Array(array=w63, index="Network") -> (element=w60:string)
        n73 = call <userlib>:"Connect.vi"("error in (no error)"=w62, "SSID"=w60) -> ("error out"=w65:errorcluster, "Feedback"=→"Log Window":string)  [unwired: 8 in]
      }
    }
    n74 = global write "Global Stop Variable.vi" "Stop"("STOP") -> ()
    n75 = Or(x=w48, y="STOP") -> (x .or. y?=w34:bool)
    n76 = Or(x=w34, y=w32) -> (x .or. y?=w33:bool)
    n77 = Or(x=w33, y=w42) -> (x .or. y?=w41:bool)
    "Color Box 3" <- w37
    "Color Box 5" <- w36
    "Color Box 4" <- w36
  }
  n78 = invoke on="Mode" class="RadioBtnsControl (strict)" method="Reinit To Default"(error in=w10) -> (error out=w9:errorcluster)  [unwired: 2 in, 2 out]
  n79 = local write "Finish"(w11) -> ()
  n80 = local write "Downloading"(w7) -> ()
  n81 = local write "Show File in Explorer"(w8) -> ()
  n82 = local write "Selesai Download"(w6) -> ()
  n83 = local write "Error"(w5) -> ()
  n84 = VISA Close(VISA resource name=w18) -> ()  [unwired: 1 in, 1 out]
  n85 = call <vilib>:"Simple Error Handler.vi"("error in (no error)"=w13) -> ()  [unwired: 4 in, 5 out]
  n86 = call <vilib>:"Simple Error Handler.vi"("error in (no error)"=w3) -> ()  [unwired: 4 in, 5 out]
  n87 = local write "STOP"(w12) -> ()
  n88 = call <vilib>:"Simple Error Handler.vi"("error in (no error)"=w9) -> ()  [unwired: 4 in, 5 out]
